vi "Finish Scan.vi"(7 "Scan finished successfully?":bool, 8 "error in":errorcluster, 11 "Scan Driver.lvclass in":refnum<class "Scan Driver.lvclass">) -> (0 "error out":errorcluster, 3 "Scan Driver.lvclass out":refnum<class "Scan Driver.lvclass">)   [LabVIEW 2009, in "Scan Driver.lvclass"]
doc: "Reset the scan and all Scanners and Readers. Write the data file. Prepare to scan again if more than one scan is requested."
uses:
  Scan Driver.lvclass
  Global/Relative Sound Files.vi
  Scan Driver.lvclass/Scan Driver.ctl
  Scanners/Scanner/Scanner.lvclass
  Readers/Reader/Reader.lvclass
  File IO/File IO.lvclass
  <vilib>/Utility/xml.llb/Write to XML File(string).vi
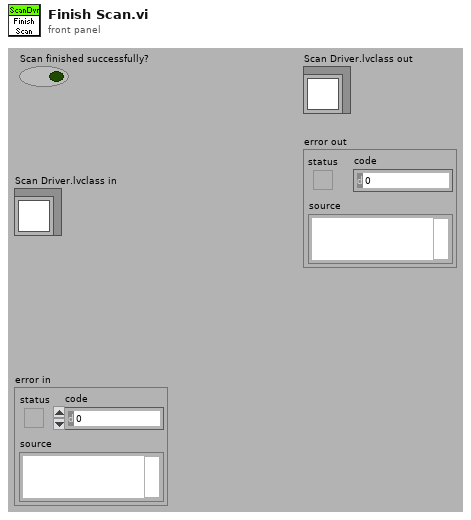
[diagram p1: front panel]
types:
  T1 = typedef "Readable.lvclass/Data Store.ctl" = T2[][]
  T2 = typedef "Readable.lvclass/Data Point.ctl" = cluster{"t":T3, "x":T4}
  T3 = typedef "Readable.lvclass/Time.ctl" = timestamp
  T4 = typedef "Readable.lvclass/X.ctl" = dbl
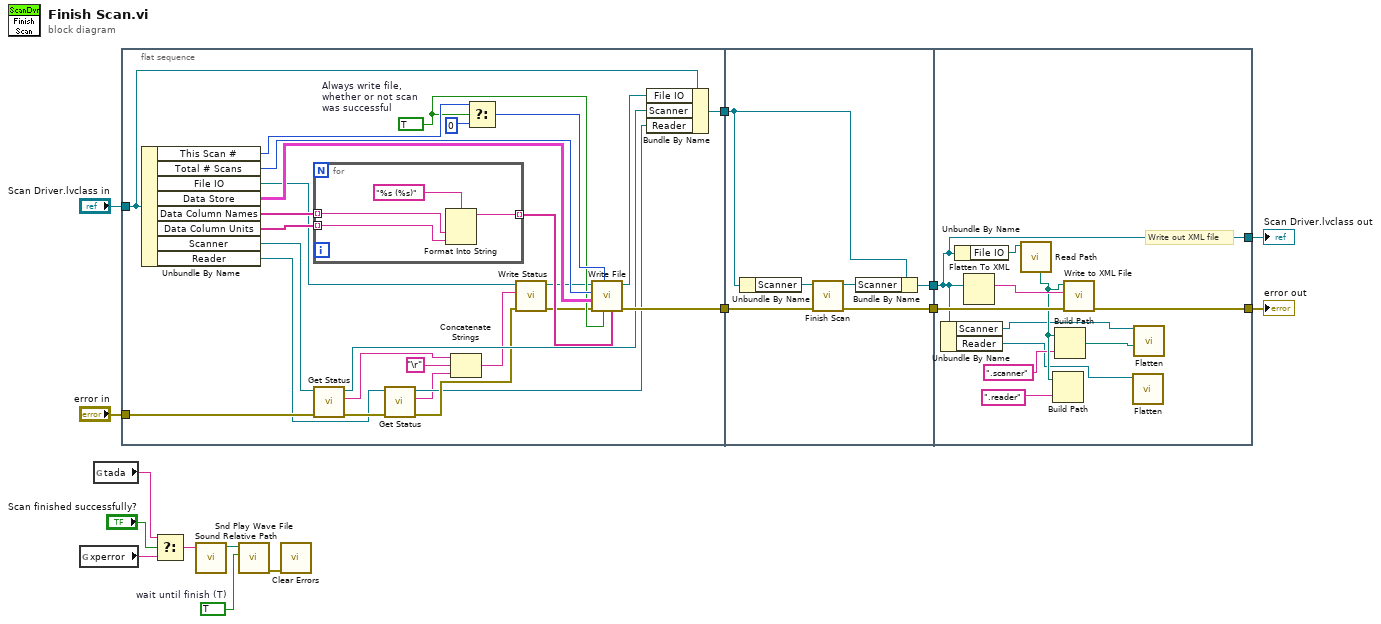
[diagram p0: block diagram]
diagram:
  w6 = TRUE  # wait until finish (T)
  n1 = global read "Relative Sound Files.vi" "xperror"() -> (w3:string)
  n2 = global read "Relative Sound Files.vi" "tada"() -> (w4:string)
  n3 = flat-sequence {
    tunnel: "error in" -> [w28]
    tunnel: "Scan Driver.lvclass in" -> [w36]
    tunnel: [w35] -> w11
    tunnel: [w34] -> w10
    tunnel: w11 -> [w50]
    tunnel: w10 -> [w49]
    tunnel: [w48] -> w9
    tunnel: [w47] -> w8
    tunnel: [w61] -> w15
    tunnel: [w57] -> w13
    tunnel: w9 -> [w57]
    tunnel: w8 -> [w60]
    frame #0 {
      w30 = TRUE  # Always write file, whether or not scan  was successful
      n4 = Unbundle By Name(w36) -> ("This Scan #"=w38:u32, "Total # Scans"=w37:u32, "File IO"=w26:refnum<class "File IO.lvclass">, "Data Store"=w41:T1, "Data Column Names"=w32:string[], "Data Column Units"=w33:string[], "Scanner"=w29:refnum<class "Scanner.lvclass">, "Reader"=w21:refnum<class "Reader.lvclass">)
      n5 = for {
        tunnel: w33 -> [w45] mode=indexing
        tunnel: w32 -> [w44] mode=indexing
        tunnel: [w43] -> w31 mode=indexing
        n6 = Format Into String(format string="%s (%s)", w44, w45) -> (resulting string=w43:string)  [unwired: 2 in, 1 out]
      }
      n7 = call "Get Status.vi"("error in (no error)"=w28, "Scanner.lvclass in"=w29) -> ("error out"=w22:errorcluster, "Status"=w17:string, "Scanner.lvclass out"=w27:refnum<class "Scanner.lvclass">)  [unwired: 7 in]
      n8 = call "Get Status.vi"("error in (no error)"=w22, "Reader.lvclass in"=w21) -> ("error out"=w23:errorcluster, "Status"=w18:string, "Reader.lvclass out"=w20:refnum<class "Reader.lvclass">)  [unwired: 7 in]
      n9 = Concatenate Strings(w17, "\r", w18) -> (w19:string)
      n10 = Select(t=w38, s=w30, f=0) -> (s? t:f=w39:u32)
      n11 = call "Write Status.vi"("error in"=w23, "Status in"=w19, "File IO.lvclass in"=w26) -> ("error out"=w24:errorcluster, "File IO.lvclass out"=w25:refnum<class "File IO.lvclass">)  [unwired: 7 in]
      n12 = call "Write File.vi"("Data Column Headings"=w31, "Write Last Run? (F)"=w30, "Current Scan #"=w39, "error in"=w24, "Data Store"=w41, "#scans"=w37, "File IO in"=w25) -> ("errorOUT"=w34:errorcluster, "File IO out"=w40:refnum<class "File IO.lvclass">)  [unwired: 3 out]
      n13 = Bundle By Name(cluster=w36, "File IO"=w40, "Scanner"=w27, "Reader"=w20) -> (w35:refnum<class "Scan Driver.lvclass">)
    }
    frame #1 {
      n14 = Unbundle By Name(w50) -> ("Scanner"=w52:refnum<class "Scanner.lvclass">)
      n15 = call-dynamic "Finish Scan.vi"("error in (no error)"=w49, "Scanner in"=w52) -> ("error out"=w47:errorcluster, "Scanner out"=w51:refnum<class "Scanner.lvclass">)  [unwired: 8 out]
      n16 = Bundle By Name(cluster=w50, "Scanner"=w51) -> (w48:refnum<class "Scan Driver.lvclass">)
    }
    frame #2 {
      # "Write out XML file"
      n17 = Unbundle By Name(w57) -> ("Scanner"=w54:refnum<class "Scanner.lvclass">, "Reader"=w53:refnum<class "Reader.lvclass">)
      n18 = Unbundle By Name(w57) -> ("File IO"=w62:refnum<class "File IO.lvclass">)
      n19 = Flatten To XML(anything=w57) -> (xml string=w63:string)
      n20 = call-dynamic "Read Path.vi"("File IO.lvclass in"=w62) -> ("Settings Path"=w59:path)  [unwired: 1 in, 9 out]
      n21 = Build Path(base path=w59, name or relative path=".reader") -> ()  [unwired: 1 out]
      n22 = Build Path(base path=w59, name or relative path=".scanner") -> (appended path=w55:path)
      n23 = call-poly <vilib>:"Write to XML File.vi"("error in (no error)"=w60, "XML Input"=w63, "XML File Path"=w59) -> ("error out"=w61:errorcluster)  [unwired: 2 in, 6 out]
      n24 = call-dynamic "Flatten.vi"("Reader in"=w53) -> ()  [unwired: 9 in, 2 out]
      n25 = call-dynamic "Flatten.vi"("Path"=w55, "Scanner in"=w54) -> ()  [unwired: 8 in, 2 out]
    }
  }
  n26 = Select(t=w4, s="Scan finished successfully?", f=w3) -> (s? t:f=w2:string)
  n27 = call "Sound Relative Path.vi"("Sound"=w2) -> ("Relative Path"=w1:path)  [unwired: 10 in]
  n28 = call <vilib>:"Snd Play Wave File.vi"("wait until finish (T)"=w6, "wave file path"=w1) -> ("error out"=w7:errorcluster)  [unwired: 1 in, 8 out]
  n29 = call <vilib>:"Clear Errors.vi"("error in (no error)"=w7) -> ()  [unwired: 7 out]
  "error out" <- w15
  "Scan Driver.lvclass out" <- w13
